vi "Refresh Hardware.vi"(8 "error in (no error)":errorcluster, 11 "HardwareHTTPController in":refnum<class "HardwareHTTPController.lvclass">) -> (0 "error out":errorcluster, 2 "Response":refnum<class "Response.lvclass">, 3 "HardwareHTTPController out":refnum<class "HardwareHTTPController.lvclass">)   [LabVIEW 2023, in "Volatus.lvlib" / "HardwareHTTPController.lvclass"]
uses:
  HardwareHTTPController.lvclass
  lv-http-util/HTTP Utils/Response/Response.lvclass
  HardwareHTTPController.lvclass/HardwareHTTPController.ctl
  MessageQ/MessageQ.lvclass/MessageQ.ctl
  MessageQ/MessageQ.lvclass
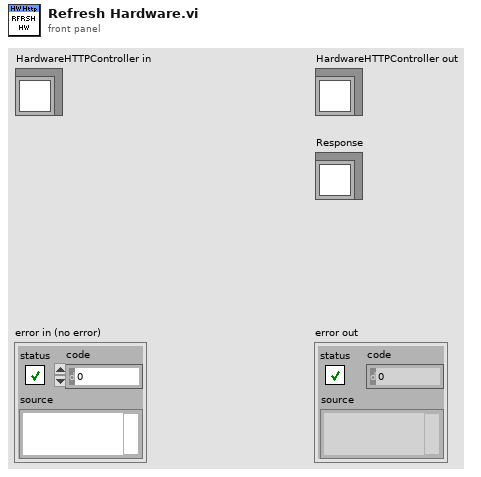
[diagram p1: front panel]
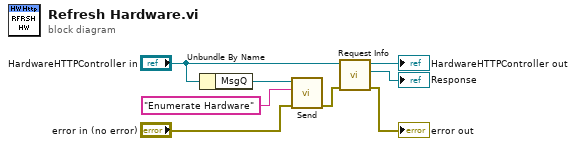
[diagram p0: block diagram]
diagram:
  n1 = Unbundle By Name("HardwareHTTPController in") -> ("MsgQ"=w6:refnum<class "MessageQ.lvclass">)
  n2 = call "Send.vi"("error in (no error)"="error in (no error)", "ID"="Enumerate Hardware", "MessageQ in"=w6) -> ("error out"=w4:errorcluster)  [unwired: 7 in, 1 out]
  n3 = call "Request Info.vi"("error in (no error)"=w4, "HardwareHTTPController in"="HardwareHTTPController in") -> ("error out"=→"error out":errorcluster, "Response"=→"Response":refnum<class "Response.lvclass">, "HardwareHTTPController out"=→"HardwareHTTPController out":refnum<class "HardwareHTTPController.lvclass">)  [unwired: 7 in]
